vi "open.vi"(8 "error in (no error)":errorcluster, 11 "filename":string) -> (0 "error out":errorcluster, 2 "ppDb out":dbl, 3 "function return":i32)   [LabVIEW 2020, in "sqlite3.lvlib"]
doc: "SQLITE_API int sqlite3_open(\n const char *filename, \n sqlite3 **ppDb \n);"
uses:
  sqlite3.lvlib
  errstr.vi
  bin/sqlite3_64.dll
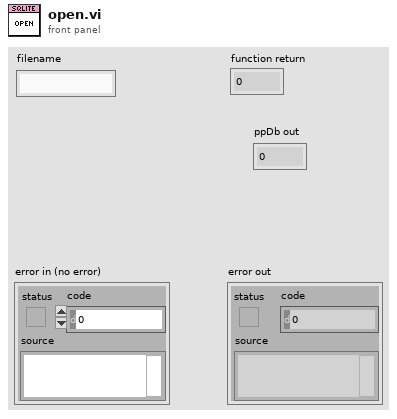
[diagram p1: front panel]
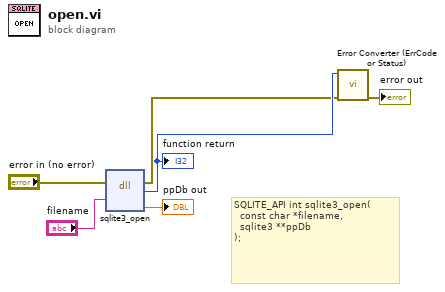
[diagram p0: block diagram]
diagram:
  # "SQLITE_API int sqlite3_open(\n  const char *filename,   \n  sqlite3 **ppDb          \n);"
  n1 = dll-call lib="C:/Users/Fred.Guo/Desktop/Database-configuration/externals/sqlite3/Source/bin/sqlite3_*.*" fn="sqlite3_open"(error in="error in (no error)", "filename"="filename") -> (error out=w3:errorcluster, w6:i32, "ppDb out"=→"ppDb out":dbl)  [unwired: 4 in, 1 out]
  "function return" <- w6
  n2 = call "Error Converter (ErrCode or Status).vi"("error in (no error)"=w3, "error code"=w6) -> ("error out"=→"error out":errorcluster)  [unwired: 9 in]
